vi "Flush.vi"(8 "Error In":errorcluster, 11 "Writer In":refnum<class "Abstract.lvclass">) -> (0 "Error Out":errorcluster, 3 "Writer Out":refnum<class "Abstract.lvclass">)   [LabVIEW 2018, in "Toolkit.lvlib" / "Writers.lvlib" / "Abstract.lvclass"]
uses:
  Abstract.lvclass
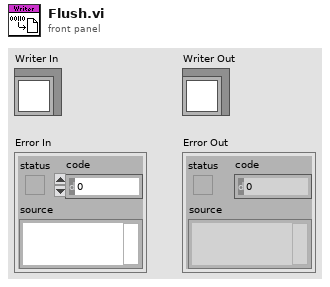
[diagram p1: front panel]
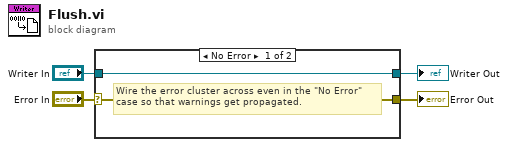
[diagram p0: block diagram]
diagram:
  n1 = case shown="No Error" "Error In" {
    selector: "Error In" -> [w5 w8]
    tunnel: [w5 w8] -> w3
    tunnel: [w6 w7] -> w1
    tunnel: "Writer In" -> [w6 w7]
    frame No Error {
      # "Wire the error cluster across even in the \"No Error\"\ncase so that warnings get propagated."
    }
    frame Error {
    }
  }
  "Error Out" <- w3
  "Writer Out" <- w1
